vi "Joints limitation.vi"(0 "joints":dbl[](array[numeric])) -> (1 "joints_limit":dbl[](array[numeric]), 2 "In Range?":bool)   [LabVIEW 2018]
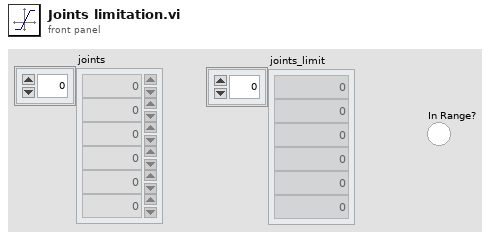
[diagram p1: front panel]
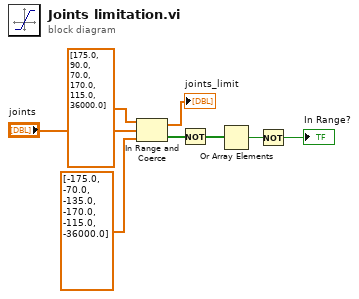
[diagram p0: block diagram]
diagram:
  n1 = In Range and Coerce(upper limit=dbl[] [175.0, 90.0, 70.0, 170.0, 115.0, 36000.0], x="joints", lower limit=dbl[] [-175.0, -70.0, -135.0, -170.0, -115.0, -36000.0] ("upper limit")) -> (coerced(x)=→"joints_limit":dbl[], In Range?=w3:bool[])
  n2 = Not(x=w3) -> (.not. x?=w2:bool[])
  n3 = Or Array Elements(Boolean array=w2) -> (logical OR=w4:bool)
  n4 = Not(x=w4) -> (.not. x?=→"In Range?":bool)
